vi "Rotate Lockin Phase.vi"(9 "Phase":dbl(slide)=67.07142639160156 step=0.5 scale=-180.0..180.0, 10 "Array Y in":dbl[](array[numeric]) format="%.2f", 11 "Array X in":dbl[](array[numeric]) format="%.2f") -> (2 "Array Y out":dbl[](array[numeric]) format="%.2f", 3 "Array X out":dbl[](array[numeric]) format="%.2f")   [LabVIEW 2015]
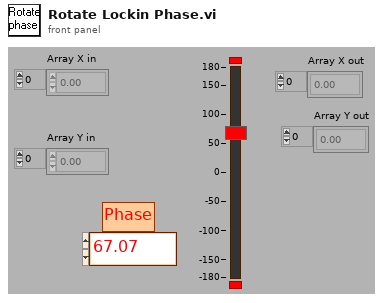
[diagram p1: front panel]
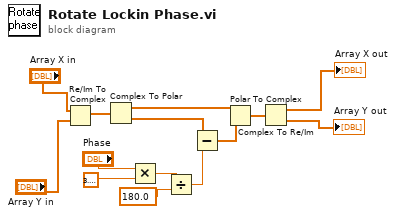
[diagram p0: block diagram]
diagram:
  n1 = Re/Im To Complex(1:"Array Y in", 2:"Array X in") -> (0:w6:cdb[])
  n2 = Complex To Polar(r * e^(i*theta)=w6) -> (r=w13:dbl[], theta=w10:dbl[])
  n3 = Multiply(x="Phase", y=3.141592653589793) -> (x*y=w8:dbl)
  n4 = Divide(x=w8, y=180.0) -> (x/y=w11:dbl)
  n5 = Subtract(x=w10, y=w11) -> (x-y=w12:dbl[])
  n6 = Polar To Complex(1:w12, 2:w13) -> (0:w14:cdb[])
  n7 = Complex To Re/Im(x + iy=w14) -> (x=→"Array X out":dbl[], y=→"Array Y out":dbl[])
